vi "File Dialog.vi"() -> (1 "Cancel Out":bool, 2 "File Name Out":path)   [LabVIEW 2022 SP3]
panel:
  in  "Cancel":bool
  in  "OK":bool
  in  "File name":path
  # "Please enter the file name"
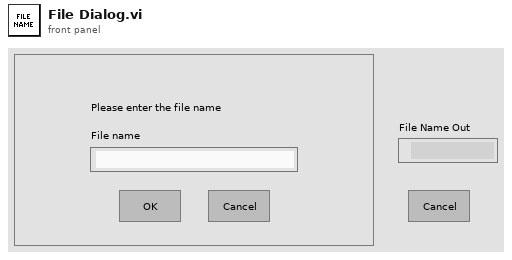
[diagram p1: front panel]
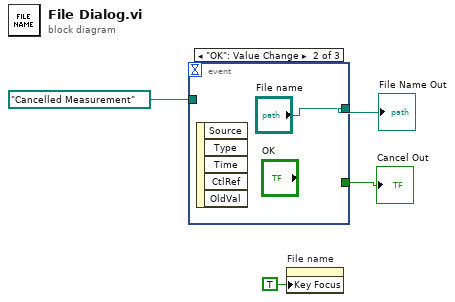
[diagram p0: block diagram]
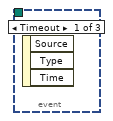
[diagram p2: hidden frame]
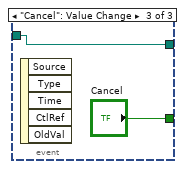
[diagram p3: hidden frame]
diagram:
  n1 = event shown="[1] \"OK\": Value Change" {
    selector: _ -> [_ _ _]
    dyn-events: _ -> [_ _ _]
    timeout: _ -> [_ _ _]
    tunnel: [_ "File name" w7] -> w4
    tunnel: path "Cancelled Measurement" -> [_ _ w7]
    tunnel: [_ _ "Cancel"] -> w2
    event Timeout {
      n2 = event-data() -> ()  [unwired: 1 in, 3 out]
    }
    event "OK": Value Change {
      n3 = event-data() -> ()  [unwired: 1 in, 5 out]
    }
    event "Cancel": Value Change {
      n4 = event-data() -> ()  [unwired: 1 in, 5 out]
    }
  }
  "File Name Out" <- w4
  "Cancel Out" <- w2
  n5 = property on="File name" class="Path"("Key Focus"=TRUE) -> ()  [unwired: 2 in, 2 out]
